vi "Read Input Level.vi"(8 "error in":errorcluster, 11 "Electronic Load in":refnum<class "Electronic Load.lvclass">) -> (0 "error out":errorcluster, 2 "Input Level":dbl, 3 "Electronic Load out":refnum<class "Electronic Load.lvclass">)   [LabVIEW 2019, in "Electronic Load.lvlib" / "Electronic Load.lvclass"]
uses:
  Library/Electronic Load.lvclass
  Library/Electronic Load.lvclass/Electronic Load.ctl
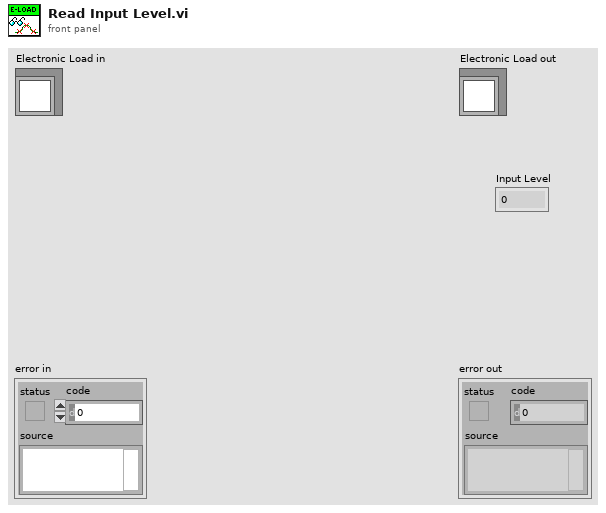
[diagram p1: front panel]
types:
  T1 = typedef "Electronic Load.lvlib/Electronic Load.lvclass/E-Load Function.ctl" = cluster{"Mode":T2, "Input Level":dbl, "Output":bool, "Slew Rate":dbl}
  T2 = typedef "Electronic Load.lvlib/Electronic Load.lvclass/E-Load Mode.ctl" = enum16{"Current", "Resistance", "Voltage"}
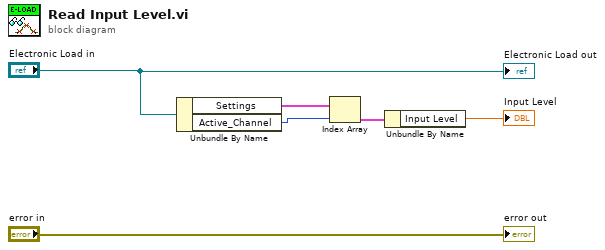
[diagram p0: block diagram]
diagram:
  n1 = Unbundle By Name("Electronic Load in") -> ("Settings"=w4:T1[], "Active_Channel"=w3:u32)
  n2 = Index Array(array=w4, index=w3) -> (element=w2:T1)
  n3 = Unbundle By Name(w2) -> ("Input Level"=→"Input Level":dbl)
  "error out" <- "error in"
  "Electronic Load out" <- "Electronic Load in"
